vi "rotg - Givens Rotation Parameters.vi"   [LabVIEW 2017, in "NI_AALBLAS.lvlib"]
doc: "Creates the parameters used in the rot - Givens Rotation VI."
uses:
  NI_AALBLAS.lvlib
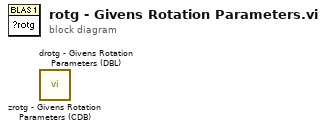
[diagram p0: block diagram]
diagram:
  n1 = call "zrotg - Givens Rotation Parameters (CDB).vi"() -> ()  [unwired: 7 in, 5 out]
  n2 = call "drotg - Givens Rotation Parameters (DBL).vi"() -> ()  [unwired: 7 in, 5 out]
